vi "Get Super String.vi"() -> ()   [LabVIEW 2024]
panel:
  out "x-y":dbl format="%#_6p"
  out "r-l diagonals":string
  out "l-r diagonals":string
  out "#diagonals":i32
  in  "Random Word Search Grid 2":string[][](array[string])=array300x300[90000 elements]
  in  "Word Search Grid":string[][](array[string])=[["R", "B", "L", "U", "E", "W"], ["E", "G", "N", "A", "R", "O"], ["D", "B", "C", "E", "W", "L"], ["L", "L", "D", "K", "V", "L"], ["P", "U", "R", "P", "L", "E"], ["N", "E", "E", "R", "G", "Y"]]
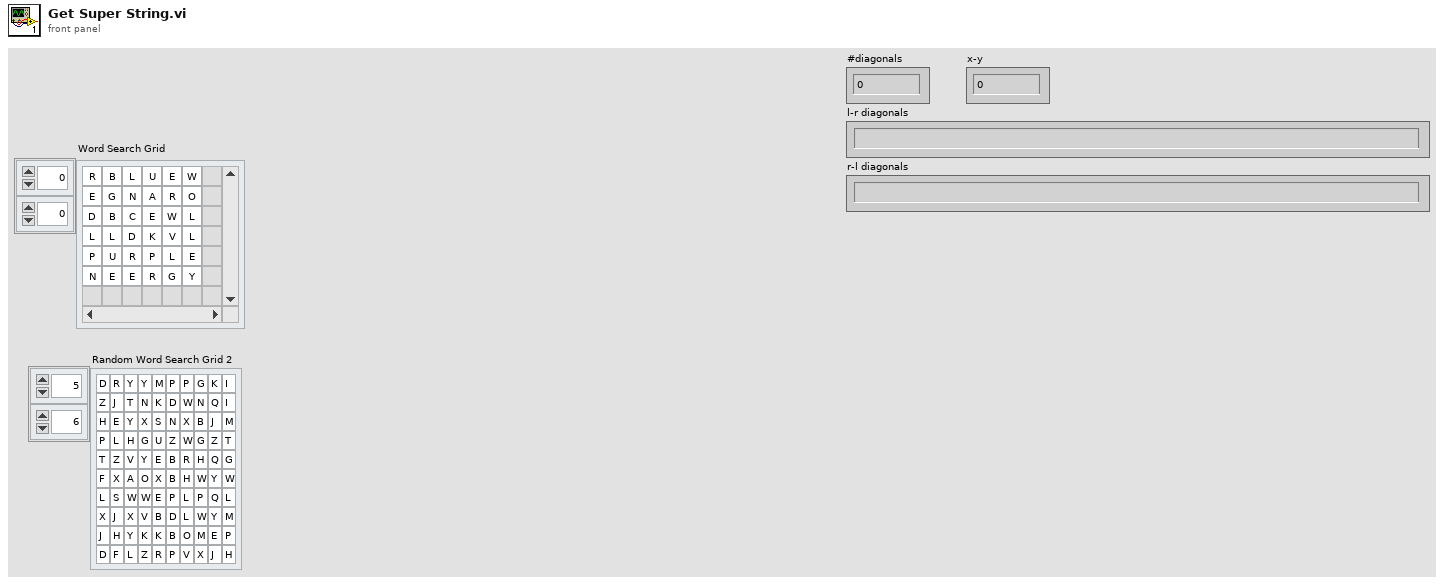
[diagram p1: front panel]
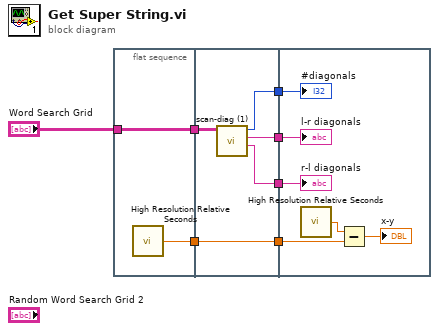
[diagram p0: block diagram]
diagram:
  n1 = flat-sequence {
    tunnel: "Word Search Grid" -> [w9]
    tunnel: [w9] -> w7
    tunnel: [w8] -> w3
    tunnel: w7 -> [w14]
    tunnel: [w13] -> w6
    tunnel: [w12] -> w5
    tunnel: [w11] -> w4
    tunnel: w3 -> [w10]
    tunnel: [w10] -> w2
    tunnel: w6 -> [w20]
    tunnel: w5 -> [w19]
    tunnel: w4 -> [w18]
    tunnel: w2 -> [w16]
    frame #0 {
      n2 = call <vilib>:"High Resolution Relative Seconds.vi"() -> ("relative seconds"=w8:dbl)
    }
    frame #1 {
      n3 = call "scan-diag (1).vi"("Word Search Grid"=w14) -> ("r-l diagonals"=w11:string, "l-r diagonals"=w12:string, "#diagonals"=w13:i32)  [unwired: 8 in]
    }
    frame #2 {
      n4 = call <vilib>:"High Resolution Relative Seconds.vi"() -> ("relative seconds"=w17:dbl)
      n5 = Subtract(x=w17, y=w16) -> (x-y=→"x-y":dbl)
      "#diagonals" <- w20
      "l-r diagonals" <- w19
      "r-l diagonals" <- w18
    }
  }
